vi "Run.vi"(8 "error in (no error)":errorcluster caption="entrée d'erreur (pas d'erreur)", 9 "labels_pred":string[][](array[string]), 10 "labels_true":string[][](array[string]), 11 "Mutual_Info_Score.lvclass":refnum<class "Mutual_Info_Score.lvclass">) -> (0 "error out":errorcluster caption="sortie d'erreur", 2 "String Data":string, 3 "Mutual_Info_Score.lvclass":refnum<class "Mutual_Info_Score.lvclass">)   [LabVIEW 2020, in "Mutual_Info_Score.lvclass"]
doc: "Returns : \n\n- mi : float\nMutual information, a non-negative value"
uses:
  Mutual_Info_Score.lvclass
  Mutual_Info_Score.lvclass/Mutual_Info_Score.ctl
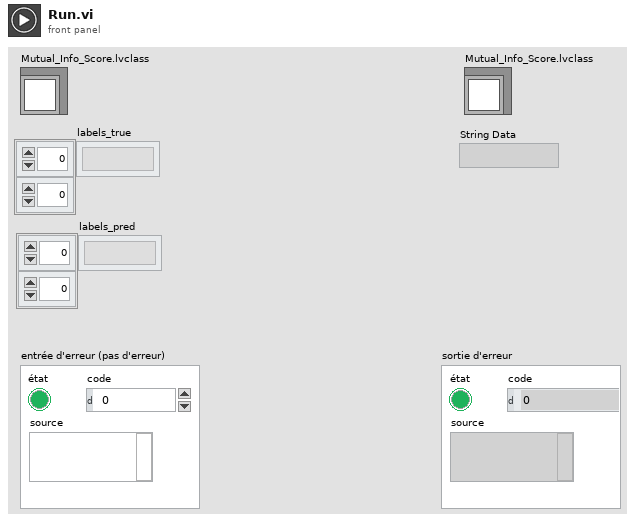
[diagram p1: front panel]
types:
  T1 = enum16{"Numeric Array", "String Array", "Sparse"}
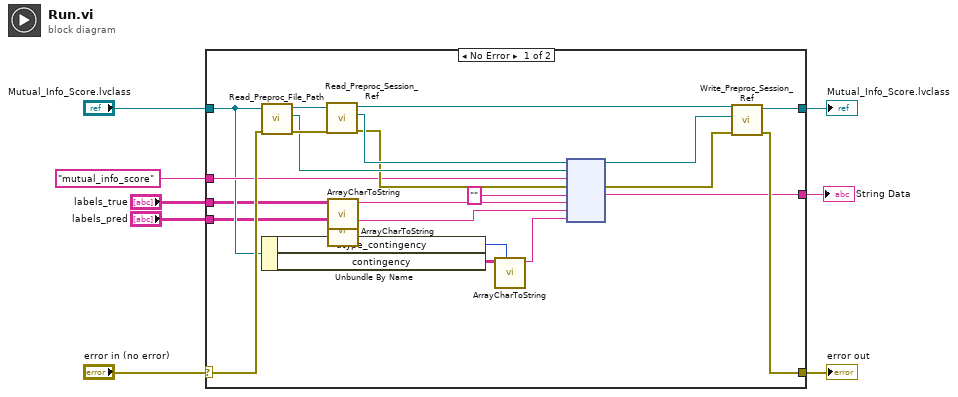
[diagram p0: block diagram]
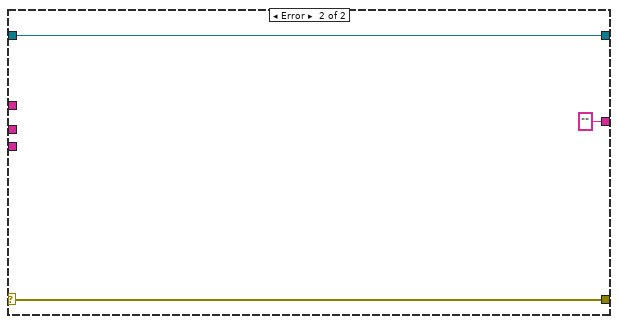
[diagram p2: hidden frame]
diagram:
  n1 = case shown="No Error" "error in (no error)" {
    selector: "error in (no error)" -> [w19 w33]
    tunnel: [w20 w33] -> w7
    tunnel: [w21 w32] -> w5
    tunnel: "Mutual_Info_Score.lvclass" -> [w16 w32]
    tunnel: "mutual_info_score" -> [w18 _]
    tunnel: [w17 ""] -> w4
    tunnel: "labels_true" -> [w12 _]
    tunnel: "labels_pred" -> [w11 _]
    frame No Error {
      n2 = call-dynamic "Read_Preproc_File_Path.vi"("error in (no error)"=w19, "Python in"=w16) -> ("error out"=w29:errorcluster, "File_Path"=w28:path, "Python out"=w30:refnum<class "Mutual_Info_Score.lvclass">)  [unwired: 7 in]
      n3 = Unbundle By Name(w16) -> ("dtype_contingency"=w15:T1, "contingency"=w14:string[][])
      n4 = call-dynamic "Read_Preproc_Session_Ref.vi"("error in (no error)"=w29, "Python in"=w30) -> ("error out"=w26:errorcluster, "Session_ref"=w27:refnum<k35>, "Python out"=w25:refnum<class "Mutual_Info_Score.lvclass">)  [unwired: 7 in]
      n5 = call "ArrayCharToString.vi"("TAB"=w12) -> ("Instruction"=w10:string)  [unwired: 10 in]
      n6 = call "ArrayCharToString.vi"("TAB"=w11) -> ("Instruction"=w9:string)  [unwired: 10 in]
      n7 = call "ArrayCharToString.vi"("Type"=w15, "TAB"=w14) -> ("Instruction"=w13:string)  [unwired: 9 in]
      n8 = node(w27, w28, w18, w26, "", w10, w9, w13) -> (w23:refnum<k35>, w24:errorcluster, w17:string)  [unwired: 3 in, 2 out]
      n9 = call-dynamic "Write_Preproc_Session_Ref.vi"("error in (no error)"=w24, "Session_ref"=w23, "Python in"=w25) -> ("error out"=w20:errorcluster, "Python out"=w21:refnum<class "Mutual_Info_Score.lvclass">)  [unwired: 7 in]
    }
    frame Error {
    }
  }
  "error out" <- w7
  "Mutual_Info_Score.lvclass" <- w5
  "String Data" <- w4
